vi "TIFF-Append Tag.vi"(0 "IFD in":u8[](array[numeric]), 5 "[IN] TagID":u16, 7 "[IN] DataType":u16(ring)=4 items=["BYTE"=1, "ASCII"=2, "SHORT"=3, "LONG"=4, "RATIONAL"=5], 9 "[IN] Data":u32[](array[numeric]), 11 "error IN":errorcluster, 12 "[IN] Byte order":T1(ring)) -> (4 "IFD out":u8[](array[numeric]), 15 "error OUT":errorcluster)   [LabVIEW 2020]
doc: "This VI writes a tif TAG. Input data is an array of U32. Note that the data should not be larger than 4 bytes."
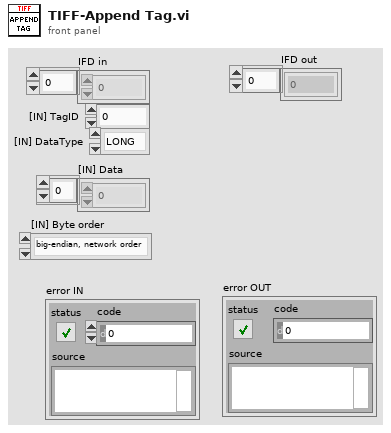
[diagram p1: front panel]
types:
  T1 = enum16{"big-endian, network order", "native, host order", "little-endian"}
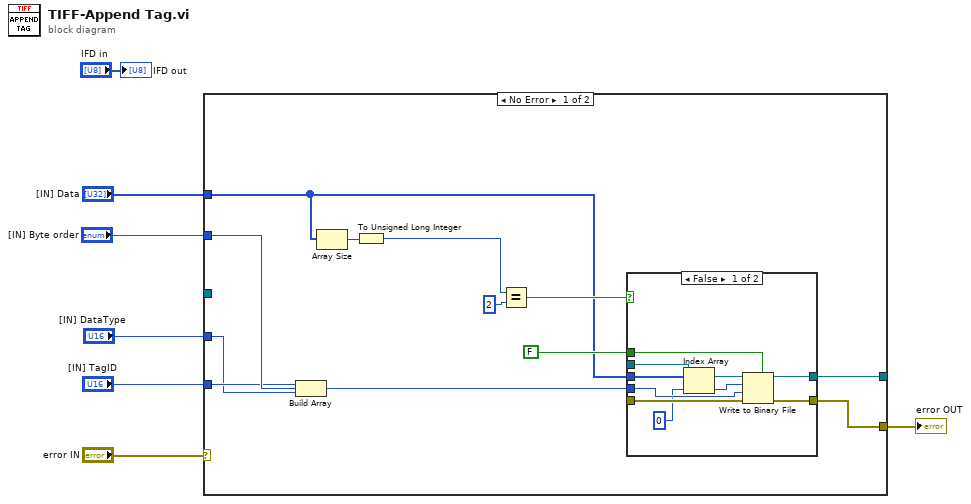
[diagram p0: block diagram]
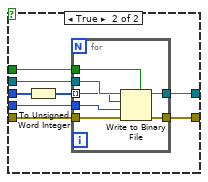
[diagram p2: hidden frame]
diagram:
  n1 = case shown="No Error" "error IN" {
    selector: "error IN" -> [_ w44]
    tunnel: _ -> [_ w45]
    tunnel: [w19 w45] -> w8
    tunnel: [w18 w44] -> w7
    tunnel: "[IN] Byte order" -> [w12 _]
    tunnel: "[IN] Data" -> [w11 _]
    tunnel: "[IN] TagID" -> [w10 _]
    tunnel: "[IN] DataType" -> [w9 _]
    frame No Error {
      n2 = Build Array(w10, w9) -> ()  [unwired: 1 out]
      n3 = Array Size(array=w11) -> (size(s)=w16:i32)
      n4 = To Unsigned Long Integer(number=w16) -> (unsigned 32bit integer=w15:u32)
      n5 = Equal?(x=w15, y=u32 2) -> (x = y?=w13:bool)
      n6 = case shown="False" w13 {
        tunnel: FALSE ("prepend array or string size? (T)") -> [w28 w36]
        tunnel: _ -> [w27 w35]
        tunnel: _ -> [w26 w34]
        tunnel: [w25 w33] -> w18
        tunnel: [w24 w32] -> w19
        tunnel: w12 -> [w23 w29]
        tunnel: w11 -> [w22 w31]
        frame False {
          n7 = Index Array(array=w22, index=0) -> (element=w21:u32)
          n8 = Write to Binary File(file (use dialog)=w26, data=w21, error in=w27, 5:w28, 9:w23) -> (refnum out=w24:refnum<file>, error out=w25:errorcluster)  [unwired: 1 in, 1 out]
        }
        frame True {
          n9 = To Unsigned Word Integer(number=w31) -> (unsigned 16bit integer=w30:u16[])
          n10 = for {
            tunnel: w36 -> [w43]
            tunnel: w30 -> [w38] mode=indexing
            tunnel: w34 -> [w41]
            tunnel: [w39] -> w32
            tunnel: w35 -> [w42]
            tunnel: [w40] -> w33
            tunnel: w29 -> [w37]
            n11 = Write to Binary File(file (use dialog)=w41, data=w38, error in=w42, 5:w43, 9:w37) -> (refnum out=w39:refnum<file>, error out=w40:errorcluster)  [unwired: 1 in, 1 out]
          }
        }
      }
    }
    frame Error {
    }
  }
  "error OUT" <- w7
  "IFD out" <- "IFD in"
